vi "FastForward.vi"(8 "Setting":T1={"P [MPa]"=0.0, "A [MPa/V]"=0.0, "P0 [MPa]"=0.0, "P start [%]"=4.0, "P end [%]"=3.5, "T0 DUT [s]"=0.0, "T0 CMBR [s]"=0.0} {"P end [%]" format="%#_13g"; "P start [%]" format="%#_13g"}, 10 "PV":dbl, 11 "SP":dbl) -> (3 "U":dbl)   [LabVIEW 2019]
uses:
  TypeDef/Setting Pressure PI.ctl
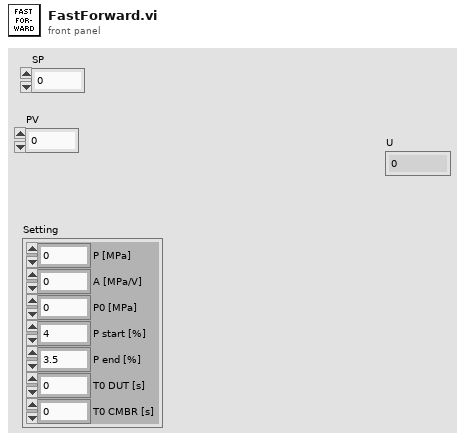
[diagram p1: front panel]
types:
  T1 = typedef "Setting Pressure PI.ctl" = cluster{"P [MPa]":dbl, "A [MPa/V]":dbl, "P0 [MPa]":dbl, "P start [%]":dbl, "P end [%]":dbl, "T0 DUT [s]":dbl, "T0 CMBR [s]":dbl}
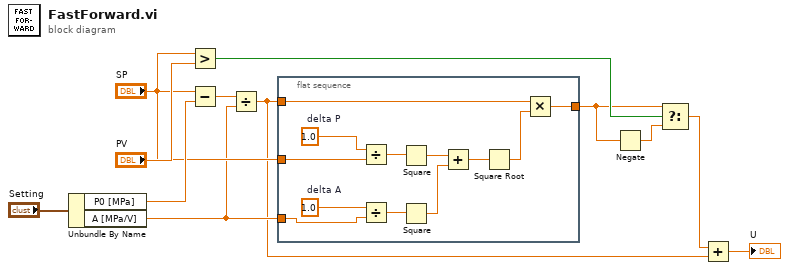
[diagram p0: block diagram]
diagram:
  n1 = Unbundle By Name("Setting") -> ("P0 [MPa]"=w11:dbl, "A [MPa/V]"=w4:dbl)
  n2 = Greater?(x="SP", y="PV") -> (0:w8:bool)
  n3 = Subtract(x="SP", y=w11) -> (x-y=w10:dbl)
  n4 = Divide(x=w10, y=w4) -> (x/y=w1:dbl)
  n5 = flat-sequence {
    tunnel: "SP" -> [w23]
    tunnel: w4 -> [w19]
    tunnel: [w14] -> w2
    tunnel: w1 -> [w13]
    frame #0 {
      w20 = 1.0  # delta A
      w24 = 1.0  # delta P
      n6 = Divide(x=w24, y=w23) -> (x/y=w22:dbl)
      n7 = Divide(x=w20, y=w19) -> (x/y=w21:dbl)
      n8 = Square(x=w22) -> (x^2=w17:dbl)
      n9 = Square(x=w21) -> (x^2=w18:dbl)
      n10 = Add(x=w17, y=w18) -> (x+y=w16:dbl)
      n11 = Square Root(x=w16) -> (sqrt(x)=w15:dbl)
      n12 = Multiply(x=w13, y=w15) -> (x*y=w14:dbl)
    }
  }
  n13 = Negate(x=w2) -> (-x=w3:dbl)
  n14 = Select(t=w2, s=w8, f=w3) -> (s? t:f=w7:dbl)
  n15 = Add(x=w7, y=w1) -> (x+y=→"U":dbl)
